vi "Runsheet.vi"(1 "Data":T1(array[cluster]), 2 "Path":string) -> ()   [LabVIEW 2017]
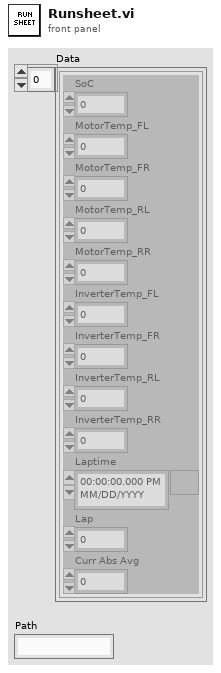
[diagram p1: front panel]
types:
  T1 = cluster{"SoC":i32, "MotorTemp_FL":dbl, "MotorTemp_FR":dbl, "MotorTemp_RL":dbl, "MotorTemp_RR":dbl, "InverterTemp_FL":dbl, "InverterTemp_FR":dbl, "InverterTemp_RL":dbl, "InverterTemp_RR":dbl, "Laptime":timestamp, "Lap":i32, "Curr Abs Avg":dbl}[]
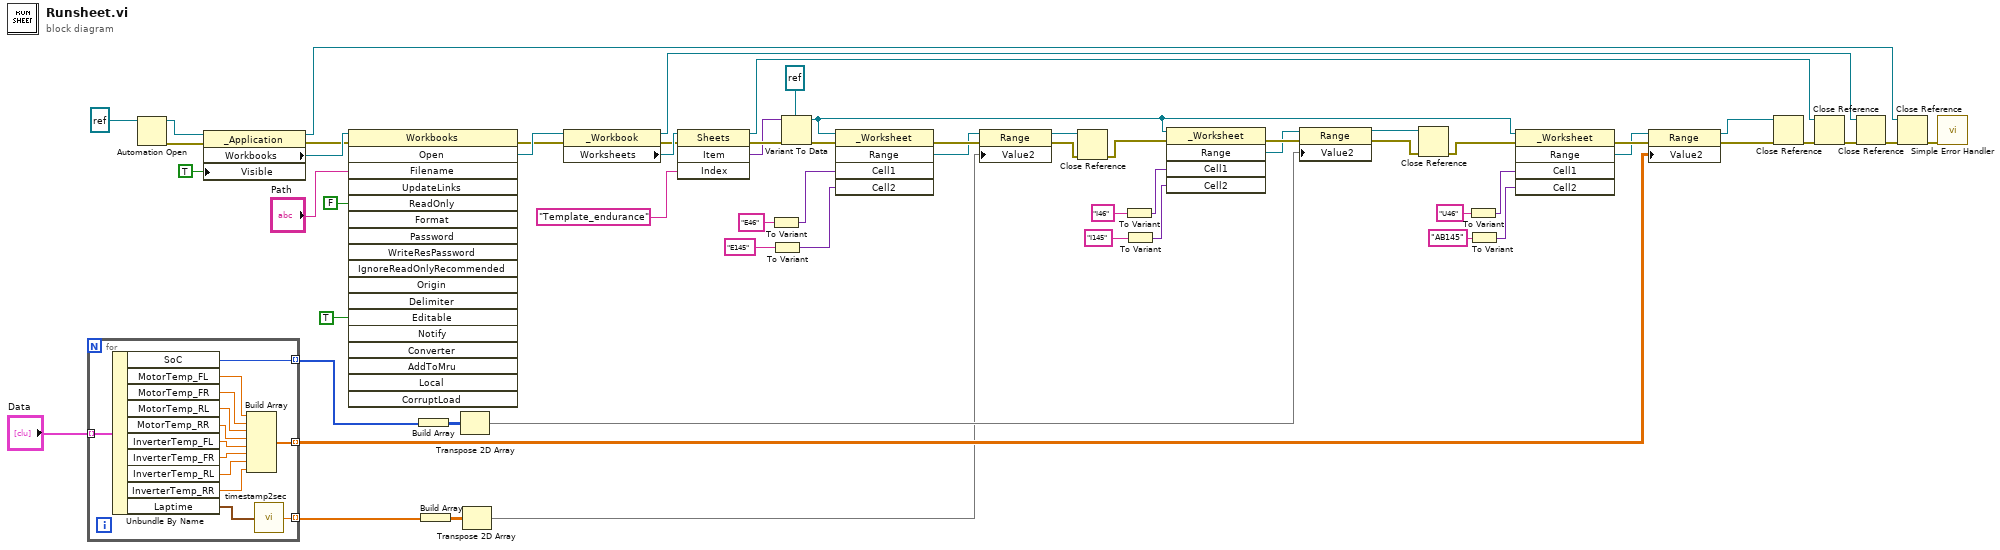
[diagram p0: block diagram]
diagram:
  n1 = for {
    tunnel: "Data" -> [w73] mode=indexing
    tunnel: [w71] -> w33 mode=indexing
    tunnel: [w70] -> w43 mode=indexing
    tunnel: [w61] -> w60 mode=indexing
    n2 = Unbundle By Name(w73) -> ("SoC"=w70:i32, "MotorTemp_FL"=w69:dbl, "MotorTemp_FR"=w68:dbl, "MotorTemp_RL"=w67:dbl, "MotorTemp_RR"=w66:dbl, "InverterTemp_FL"=w65:dbl, "InverterTemp_FR"=w64:dbl, "InverterTemp_RL"=w63:dbl, "InverterTemp_RR"=w62:dbl, "Laptime"=w72:timestamp)
    n3 = Build Array(w69, w68, w67, w66, w65, w64, w63, w62) -> (w61:dbl[])
    n4 = call "timestamp2sec.vi"("Laptime"=w72) -> ("seconds"=w71:dbl)
  }
  n5 = Automation Open(Automation Refnum=refnum<k7> refnum ("Excel._Application")) -> (Automation Refnum=w2:refnum<k7>, error out=w3:errorcluster)  [unwired: 3 in]
  n6 = property on="Property Node" class="_Application"(reference=w2, error in=w3, "Visible"=TRUE) -> (reference out=w29:refnum<k7>, error out=w7:errorcluster, "Workbooks"=w8:refnum<k7>)
  n7 = invoke on="Invoke Node" class="Workbooks" method="Open"(reference=w8, error in=w7, "Filename"="Path", "ReadOnly"=FALSE, "Editable"=TRUE) -> (error out=w12:errorcluster, "Open"=w13:refnum<k7>)  [unwired: 13 in, 16 out]
  n8 = Build Array(w43) -> (w42:i32[][])
  n9 = Build Array(w33) -> (w39:dbl[][])
  n10 = Transpose 2D Array(2D array=w42) -> (transposed array=w44:i32[][])
  n11 = Transpose 2D Array(2D array=w39) -> (transposed array=w40:dbl[][])
  n12 = property on="Property Node" class="_Workbook"(reference=w13, error in=w12) -> (reference out=w28:refnum<k7>, error out=w9:errorcluster, "Worksheets"=w11:refnum<k7>)
  n13 = invoke on="Invoke Node" class="Sheets" method="Item"(reference=w11, error in=w9, "Index"="Template_endurance" ("Name of Worksheet")) -> (reference out=w27:refnum<k7>, error out=w16:errorcluster, "Item"=w15:variant)  [unwired: 1 in, 1 out]
  n14 = To Variant(anything="E46") -> (Variant=w20:variant)
  n15 = To Variant(anything="E145") -> (Variant=w22:variant)
  n16 = Variant To Data(error in=w16, type=refnum<k7> refnum ("reference"), Variant=w15) -> (data=w51:refnum<k7>, error out=w17:errorcluster)
  n17 = invoke on="Invoke Node" class="_Worksheet" method="Range"(reference=w51, error in=w17, "Cell1"=w20, "Cell2"=w22) -> (error out=w32:errorcluster, "Range"=w31:refnum<k7>)  [unwired: 1 in, 3 out]
  n18 = property class="Range"(reference=w31, error in=w32, "Value2"=w40) -> (reference out=w57:refnum<k7>, error out=w58:errorcluster)
  n19 = Close Reference(reference=w57, error in (no error)=w58) -> (error out=w59:errorcluster)
  n20 = To Variant(anything="I46") -> (Variant=w37:variant)
  n21 = To Variant(anything="I145") -> (Variant=w38:variant)
  n22 = invoke on="Invoke Node" class="_Worksheet" method="Range"(reference=w51, error in=w59, "Cell1"=w37, "Cell2"=w38) -> (error out=w41:errorcluster, "Range"=w34:refnum<k7>)  [unwired: 1 in, 3 out]
  n23 = property class="Range"(reference=w34, error in=w41, "Value2"=w44) -> (reference out=w55:refnum<k7>, error out=w54:errorcluster)
  n24 = Close Reference(reference=w55, error in (no error)=w54) -> (error out=w56:errorcluster)
  n25 = To Variant(anything="U46") -> (Variant=w48:variant)
  n26 = To Variant(anything="AB145") -> (Variant=w49:variant)
  n27 = invoke on="Invoke Node" class="_Worksheet" method="Range"(reference=w51, error in=w56, "Cell1"=w48, "Cell2"=w49) -> (error out=w50:errorcluster, "Range"=w45:refnum<k7>)  [unwired: 1 in, 3 out]
  n28 = property class="Range"(reference=w45, error in=w50, "Value2"=w60) -> (reference out=w52:refnum<k7>, error out=w53:errorcluster)
  n29 = Close Reference(reference=w52, error in (no error)=w53) -> (error out=w26:errorcluster)
  n30 = Close Reference(reference=w27, error in (no error)=w26) -> (error out=w24:errorcluster)
  n31 = Close Reference(reference=w28, error in (no error)=w24) -> (error out=w25:errorcluster)
  n32 = Close Reference(reference=w29, error in (no error)=w25) -> (error out=w23:errorcluster)
  n33 = call <vilib>:"Simple Error Handler.vi"("error in (no error)"=w23) -> ()  [unwired: 4 in, 5 out]
